vi "inches to encoder counts.vi"(10 "x inches":dbl) -> (2 "encoder counts":dbl)   [LabVIEW 2016]
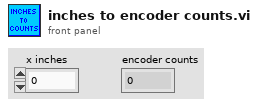
[diagram p1: front panel]
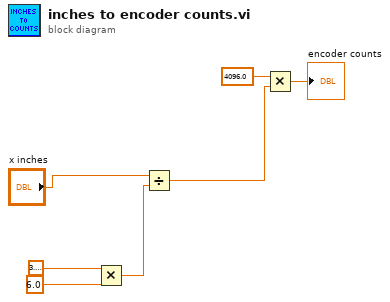
[diagram p0: block diagram]
diagram:
  n1 = Multiply(x=3.141592653589793, y=6.0) -> (x*y=w3:dbl)
  n2 = Divide(x="x inches", y=w3) -> (x/y=w2:dbl)
  n3 = Multiply(x=4096.0, y=w2) -> (x*y=→"encoder counts":dbl)
